vi "Teleop.vi"(10 "Match Info":T1={"Autonomous Elapsed Seconds"=0.0, "TeleOp Elapsed Seconds"=0.0, "Disabled Elapsed Seconds"=0.0, "Visited Autonomous"=FALSE, "Visited TeleOp"=FALSE, "Visited Disabled"=FALSE, "Autonomous Settings"={"Autonomous Style"=enum."Independent", "VI Refnum"=refnum}}, 11 "Call Context":T2) -> ()   [LabVIEW 2017]
doc: "This VI is called for each TeleOp packet received from the DS where the robot is not disabled. It is often used to read from the joysticks and update I/O or to update setpoints for timed control loops. It should complete and return within 20 milliseconds or it may miss DS packets."
uses:
  <vilib>/Rock Robotics/WPI/DriverStation/WPI_DriverStationDerivedRobotMode.ctl
  <vilib>/Rock Robotics/WPI/DriverStation/WPI_DriverStationMatch Info.ctl
  <vilib>/Rock Robotics/WPI/Relay/WPI_RelayValue.ctl
  <vilib>/Rock Robotics/WPI/Utilities/WPI_GetSetVariantRefNum.vi
  <vilib>/Rock Robotics/Network Tables/NT Read Boolean.vi
  <vilib>/Rock Robotics/Network Tables/NT Read Number.vi
  Robot Global Data.vi
  <vilib>/Rock Robotics/Network Tables/NT Write Number.vi
  <vilib>/Rock Robotics/Network Tables/NT Write Numeric Array.vi
panel:
  out "xout":dbl
  out "yout":dbl
  out "Sample Slider 0":dbl(slide) scale=0.0..5.0
  out "Sample Boolean 1":bool
  out "Sample Boolean 0":bool
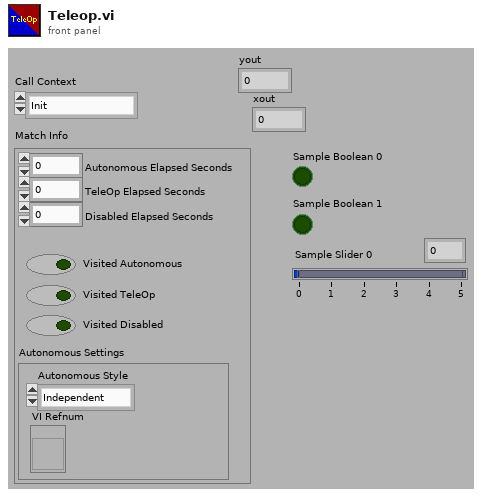
[diagram p1: front panel]
types:
  T1 = typedef "WPI_DriverStationMatch Info.ctl" = cluster{"Autonomous Elapsed Seconds":dbl, "TeleOp Elapsed Seconds":dbl, "Disabled Elapsed Seconds":dbl, "Visited Autonomous":bool, "Visited TeleOp":bool, "Visited Disabled":bool, "Autonomous Settings":cluster{"Autonomous Style":enum16{"Iterative", "Independent"}, "VI Refnum":refnum<vi>}}
  T2 = typedef "WPI_DriverStationDerivedRobotMode.ctl" = enum16{"Init", "Execute", "Stop"}
  T3 = typedef "WPI_RobotDriveDevRef.ctl" = cluster{"DevStatus":errorcluster, "Motors[]":T4[], "Square Inputs":bool, "Max Output":dbl}
  T4 = typedef "WPI_MotorControlDeviceRef.ctl" = cluster{"DeviceStatus":errorcluster, "Type":T5, "PWM":cluster{"PWM Channel":T6, "DeadBand":T7}, "CAN":cluster{"Device Number":u8, "SetOutput VI Ref":variant, "GetOutput VI Ref":variant, "Enable VI Ref":variant, "Disable VI Ref":variant, "Data":variant}, "Invert":bool, "DIO PWM":cluster{"PWM \"Enable\" Channel":T6, "DIOChannel":T8, "PWM Rate":dbl}}
  T5 = typedef "WPI_MotorControlType.ctl" = enum16{"PWM", "CAN", "DIO PWM"}
  T6 = typedef "FPGA_DIOPWMChannel.ctl" = enum8{"PWM 0", "PWM 1", "PWM 2", "PWM 3", "PWM 4", "PWM 5", "PWM 6", "PWM 7", "PWM 8", "PWM 9", "PWM MXP 0", "PWM MXP 1", "PWM MXP 2", "PWM MXP 3", "PWM MXP 4", "PWM MXP 5", "PWM MXP 6", "PWM MXP 7", "PWM MXP 8", "PWM MXP 9", "Invalid"}
  T7 = typedef "WPI_PWMDeadband.ctl" = cluster{"Name":string, "maxPositivePwm":i32, "minPositivePwm":i32, "centerPwm":i32, "maxNegativePwm":i32, "minNegativePwm":i32, "angularRange":u16}
  T8 = typedef "FPGA_DIOChannel.ctl" = enum8{"DIO 0", "DIO 1", "DIO 2", "DIO 3", "DIO 4", "DIO 5", "DIO 6", "DIO 7", "DIO 8", "DIO 9", "DIO MXP 0", "DIO MXP 1", "DIO MXP 2", "DIO MXP 3", "DIO MXP 4", "DIO MXP 5", "DIO MXP 6", "DIO MXP 7", "DIO MXP 8", "DIO MXP 9", "DIO MXP 10", "DIO MXP 11", "DIO MXP 12", "DIO MXP 13", "DIO MXP 14", "DIO MXP 15", "SPI Port CS1", "SPI Port CS2", "SPI Port CS3", "SPI Port MISO", "SPI Port MOSI", "Invalid"}
  T9 = typedef "WPI_JoystickDevRef.ctl" = cluster{"Device":T10}
  T10 = typedef "WPI_JoystickDeviceEnum.ctl" = enum16{"USB 0", "USB 1", "USB 2", "USB 3", "USB 4", "USB 5"}
  T11 = typedef "WPI_RelayValue.ctl" = enum16{"Off", "On", "Forward", "Reverse"}
  T12 = typedef "WPI_RelayDevRef.ctl" = cluster{"DevStatus":errorcluster, "Relay Channel":T13, "Relay Direction":T14}
  T13 = typedef "FPGA_DIORelayChannel.ctl" = enum8{"Relay 0", "Relay 1", "Relay 2", "Relay 3", "Invalid"}
  T14 = typedef "WPI_RelayDirection.ctl" = enum16{"Both directions", "Forward only", "Reverse only"}
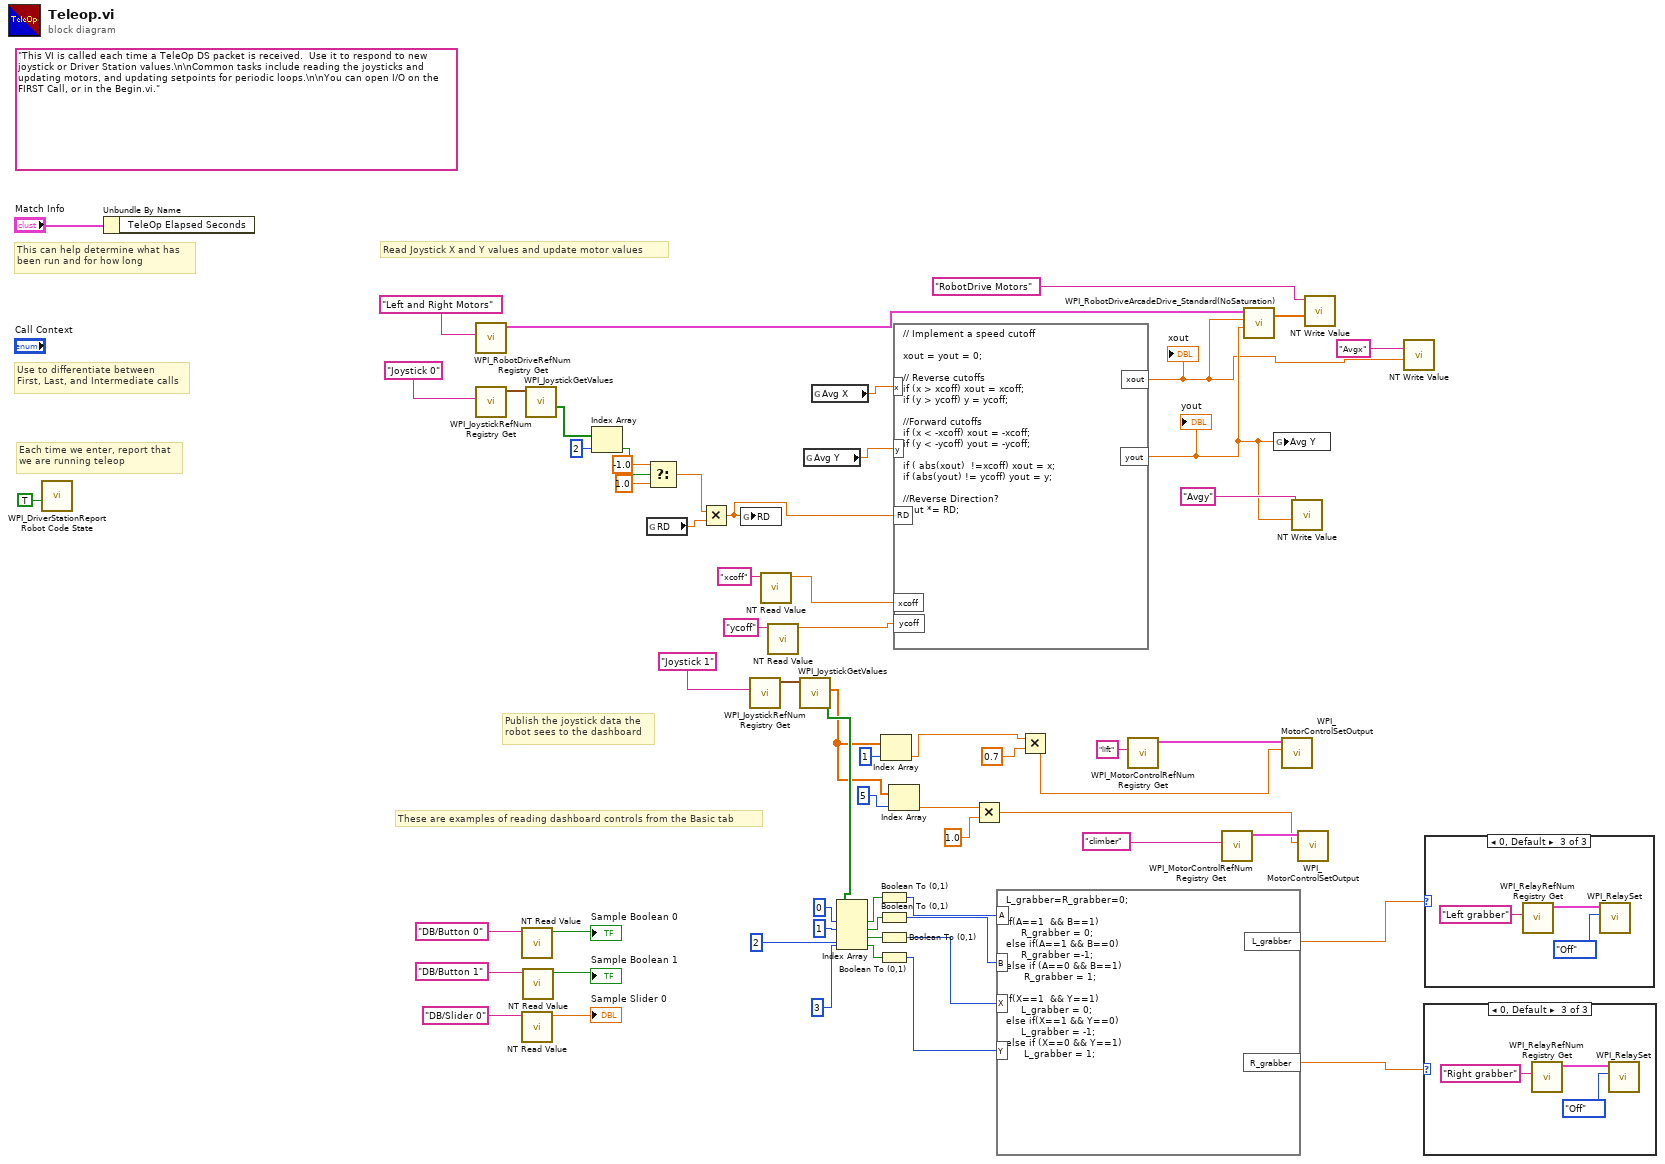
[diagram p0: block diagram]
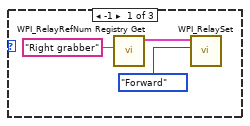
[diagram p2: hidden frame]
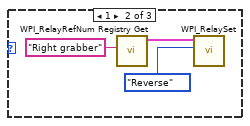
[diagram p3: hidden frame]
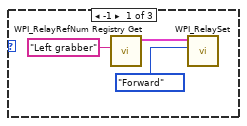
[diagram p4: hidden frame]
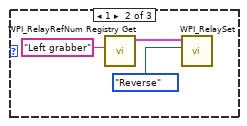
[diagram p5: hidden frame]
diagram:
  (unwired) "This VI is called each time a TeleOp DS packet is received.  Use it to respond to new joystick or Driver Station values.\n\nCommon tasks include reading the joysticks and updating motors, and updating setpoints for periodic loops.\n\nYou can open I/O on the FIRST Call, or in the Begin.vi."
  # "These are examples of reading dashboard controls from the Basic tab"
  # "Publish the joystick data the\nrobot sees to the dashboard"
  # "Each time we enter, report that\nwe are running teleop"
  # "Use to differentiate between\nFirst, Last, and Intermediate calls"
  # "This can help determine what has\nbeen run and for how long"
  # "Read Joystick X and Y values and update motor values"
  n1 = call <vilib>:"WPI_DriverStationReport Robot Code State.vi"("TeleOp"=TRUE ("Autonomous")) -> ()  [unwired: 10 in, 1 out]
  n2 = Unbundle By Name("Match Info") -> ()  [unwired: 1 out]
  n3 = call <vilib>:"WPI_RobotDriveRefNum Registry Get.vi"("refnum name"="Left and Right Motors") -> ("RobotDriveDevRef"=w49:T3)  [unwired: 1 in, 9 out]
  n4 = call <vilib>:"WPI_JoystickRefNum Registry Get.vi"("refnum name"="Joystick 0") -> ("JoystickDevRef"=w59:T9)  [unwired: 1 in, 9 out]
  n5 = call-poly <vilib>:"NT Read Value.vi"("Name"="DB/Button 0" ("refnum name")) -> ("Boolean"=→"Sample Boolean 0":bool)  [unwired: 9 in, 1 out]
  n6 = call-poly <vilib>:"NT Read Value.vi"("Name"="DB/Slider 0" ("refnum name")) -> ("Numeric"=→"Sample Slider 0":dbl)  [unwired: 9 in, 1 out]
  n7 = call-poly <vilib>:"NT Read Value.vi"("Name"="DB/Button 1" ("refnum name")) -> ("Boolean"=→"Sample Boolean 1":bool)  [unwired: 9 in, 1 out]
  n8 = call <vilib>:"WPI_JoystickGetValues.vi"("JoystickDevRef"=w59) -> ("Buttons"=w13:bool[])  [unwired: 6 in, 4 out]
  n9 = Index Array(array=w13, index=2) -> (element=w11:bool)
  n10 = global read "Robot Global Data.vi" "RD"() -> (w7:dbl)
  n11 = Select(t=-1.0, s=w11, f=1.0) -> (s? t:f=w8:dbl)
  n12 = Multiply(x=w8, y=w7) -> (x*y=w6:dbl)
  n13 = global write "Robot Global Data.vi" "RD"(w6) -> ()
  n14 = call <vilib>:"WPI_JoystickRefNum Registry Get.vi"("refnum name"="Joystick 1") -> ("JoystickDevRef"=w38:T9)  [unwired: 1 in, 9 out]
  n15 = call-poly <vilib>:"NT Read Value.vi"("Name"="xcoff") -> ("Numeric"=w4:dbl)  [unwired: 9 in, 1 out]
  n16 = call-poly <vilib>:"NT Read Value.vi"("Name"="ycoff") -> ("Numeric"=w3:dbl)  [unwired: 9 in, 1 out]
  n17 = call <vilib>:"WPI_JoystickGetValues.vi"("JoystickDevRef"=w38) -> ("Buttons"=w35:bool[], "Axes"=w21:dbl[])  [unwired: 6 in, 3 out]
  n18 = global read "Robot Global Data.vi" "Avg Y"() -> (w47:dbl)
  n19 = global read "Robot Global Data.vi" "Avg X"() -> (w48:dbl)
  n20 = Index Array(array=w35, index #1=0 ("index"), index #2=1 ("index"), index #3=2 ("index"), index #4=3 ("index")) -> (element #1=w30:bool, element #2=w26:bool, element #3=w27:bool, element #4=w28:bool)
  n21 = Boolean To (0,1)(Boolean=w30) -> (0, 1=w29:i16)
  n22 = Boolean To (0,1)(Boolean=w26) -> (0, 1=w25:i16)
  n23 = Boolean To (0,1)(Boolean=w27) -> (0, 1=w24:i16)
  n24 = Boolean To (0,1)(Boolean=w28) -> (0, 1=w23:i16)
  n25 = Index Array(array=w21, index=1) -> (element=w36:dbl)
  n26 = Index Array(array=w21, index=5) -> (element=w19:dbl)
  n27 = formula code="// Implement a speed cutoff\n\nxout = yout = 0;\n\n// Reverse cutoffs\nif (x > xcoff) xout = xcoff; \nif (y > ycoff) y = ycoff;\n\n//Forward cutoffs\nif (x < -xcoff) xout = -xcoff;\nif (y < -ycoff) yout = -ycoff;\n\nif ( abs(xout)  !=xcoff) xout = x;\nif (abs(yout) != ycoff) yout = y;\n\n//Reverse Direction?\nyout *= RD;"("x"=w48, "y"=w47, "RD"=w6, "xcoff"=w4, "ycoff"=w3) -> ("xout"=w5:dbl, "yout"=w44:dbl)
  "yout" <- w44
  "xout" <- w5
  n28 = Multiply(x=w19, y=1.0) -> (x*y=w16:dbl)
  n29 = formula code="L_grabber=R_grabber=0;\n\nif(A==1  && B==1)\n     R_grabber = 0;\nelse if(A==1 && B==0)\n     R_grabber =-1;\nelse if (A==0 && B==1)\n      R_grabber = 1;\n\nif(X==1  && Y==1)\n     L_grabber = 0;\nelse if(X==1 && Y==0)\n     L_grabber = -1;\nelse if (X==0 && Y==1)\n      L_grabber = 1;"("A"=w29, "B"=w25, "X"=w24, "Y"=w23) -> ("L_grabber"=w15:dbl, "R_grabber"=w14:dbl)
  n30 = Multiply(x=w36, y=0.7) -> (x*y=w40:dbl)
  n31 = call <vilib>:"WPI_MotorControlRefNum Registry Get.vi"("refnum name"="lift") -> ("MotorControlDevRef"=w42:T4)  [unwired: 9 in, 1 out]
  n32 = call <vilib>:"WPI_MotorControlRefNum Registry Get.vi"("refnum name"="climber") -> ("MotorControlDevRef"=w17:T4)  [unwired: 9 in, 1 out]
  n33 = call <vilib>:"WPI_RobotDriveArcadeDrive_Standard(NoSaturation).vi"("Y axis value"=w44, "X axis value"=w5, "RobotDriveDevRef"=w49) -> ("Motor Values"=w50:dbl[])  [unwired: 1 in, 7 out]
  n34 = global write "Robot Global Data.vi" "Avg Y"(w44) -> ()
  n35 = call <vilib>:"WPI_MotorControlSetOutput.vi"("Output"=w40, "MotorControlDevRef"=w42) -> ()  [unwired: 7 in, 3 out]
  n36 = call-poly <vilib>:"NT Write Value.vi"("Numeric"=w44, "Name"="Avgy") -> ()  [unwired: 9 in, 1 out]
  n37 = call <vilib>:"WPI_MotorControlSetOutput.vi"("Output"=w16, "MotorControlDevRef"=w17) -> ()  [unwired: 7 in, 3 out]
  n38 = call-poly <vilib>:"NT Write Value.vi"("Numeric Array"=w50, "Name"="RobotDrive Motors") -> ()  [unwired: 9 in, 1 out]
  n39 = call-poly <vilib>:"NT Write Value.vi"("Numeric"=w5, "Name"="Avgx") -> ()  [unwired: 9 in, 1 out]
  n40 = case shown="0, Default" w14 {
    frame -1 {
      n41 = call <vilib>:"WPI_RelayRefNum Registry Get.vi"("refnum name"="Right grabber") -> ("RelayDevRef"=w65:T12)  [unwired: 9 in, 1 out]
      n42 = call <vilib>:"WPI_RelaySet.vi"("RelayValue"=WPI_RelayValue."Forward", "RelayDevRef"=w65) -> ()  [unwired: 8 in, 2 out]
    }
    frame 1 {
      n43 = call <vilib>:"WPI_RelayRefNum Registry Get.vi"("refnum name"="Right grabber") -> ("RelayDevRef"=w68:T12)  [unwired: 9 in, 1 out]
      n44 = call <vilib>:"WPI_RelaySet.vi"("RelayValue"=WPI_RelayValue."Reverse", "RelayDevRef"=w68) -> ()  [unwired: 8 in, 2 out]
    }
    frame 0, Default {
      n45 = call <vilib>:"WPI_RelayRefNum Registry Get.vi"("refnum name"="Right grabber") -> ("RelayDevRef"=w70:T12)  [unwired: 9 in, 1 out]
      n46 = call <vilib>:"WPI_RelaySet.vi"("RelayValue"=WPI_RelayValue."Off", "RelayDevRef"=w70) -> ()  [unwired: 8 in, 2 out]
    }
  }
  n47 = case shown="0, Default" w15 {
    frame -1 {
      n48 = call <vilib>:"WPI_RelayRefNum Registry Get.vi"("refnum name"="Left grabber") -> ("RelayDevRef"=w74:T12)  [unwired: 9 in, 1 out]
      n49 = call <vilib>:"WPI_RelaySet.vi"("RelayValue"=WPI_RelayValue."Forward", "RelayDevRef"=w74) -> ()  [unwired: 8 in, 2 out]
    }
    frame 1 {
      n50 = call <vilib>:"WPI_RelayRefNum Registry Get.vi"("refnum name"="Left grabber") -> ("RelayDevRef"=w77:T12)  [unwired: 9 in, 1 out]
      n51 = call <vilib>:"WPI_RelaySet.vi"("RelayValue"=WPI_RelayValue."Reverse", "RelayDevRef"=w77) -> ()  [unwired: 8 in, 2 out]
    }
    frame 0, Default {
      n52 = call <vilib>:"WPI_RelayRefNum Registry Get.vi"("refnum name"="Left grabber") -> ("RelayDevRef"=w79:T12)  [unwired: 9 in, 1 out]
      n53 = call <vilib>:"WPI_RelaySet.vi"("RelayValue"=WPI_RelayValue."Off", "RelayDevRef"=w79) -> ()  [unwired: 8 in, 2 out]
    }
  }
